vi "Vertical Profile.vi"(5 "Vert.Z-Locations":dbl[](array[numeric])=[12.7, 19.05, 25.4], 6 "Averaging time (min)":dbl, 7 "Lat.Coords":T1={"X"=-3390.0, "Y"=-113.0, "Z"=780.0, "Name"="Anemo1", "Spacing"=enum."Specified", "start"=780.0, "end"=780.0, "NumPts"=780.0, "Specified Locns"=[]}, 9 "Direction":enum16{"Forward", "Reverse"}(ring), 10 "Tunnel Speed":dbl, 11 "Input Task Array":T2[](array[typedef]) {"Carrier_2 Q (l/min)" format="%#.2f"; "Row Duration (mins)" format="%#.1f"; "Row No" min=0; "Trace Gas Concentration (%)" min=0.0 format="%#_4f"; "Carrier_1 Q (l/min)" format="%#.2f"; "Tunnel Speed" format="%#.2f"; "Start X" format="%#.2f"; "Start Y" format="%#.2f"; "Start Z" format="%#.2f"; "End X" format="%#.2f"; "End Y" format="%#.2f"; "End Z" format="%#.2f"; "Averaging time (min)" min=0.0 format="%#.2f"}) -> (3 "Output Task Array":T2[](array[typedef]) {"Carrier_2 Q (l/min)" format="%#.2f"; "Row Duration (mins)" format="%#.1f"; "Row No" min=0; "Trace Gas Concentration (%)" min=0.0 format="%#_4f"; "Carrier_1 Q (l/min)" format="%#.2f"; "Tunnel Speed" format="%#.2f"; "Start X" format="%#.2f"; "Start Y" format="%#.2f"; "Start Z" format="%#.2f"; "End X" format="%#.2f"; "End Y" format="%#.2f"; "End Z" format="%#.2f"; "Averaging time (min)" min=0.0 format="%#.2f"})   [LabVIEW 2015]
uses:
  RowTemplate.ctl
  Anemometry Sub Vis/Gen Trav/Spacing.ctl
  Anemometry Sub Vis/Controls/Multi_run_mode.ctl
  MRCMDFBGlobal.vi
  Set ADAM Ch.vi
panel:
  out "dz":dbl
  # "X           Y            Z"
  # "Start"
  # "End"
  # "X           Y            Z"
  # "Start"
  # "End"
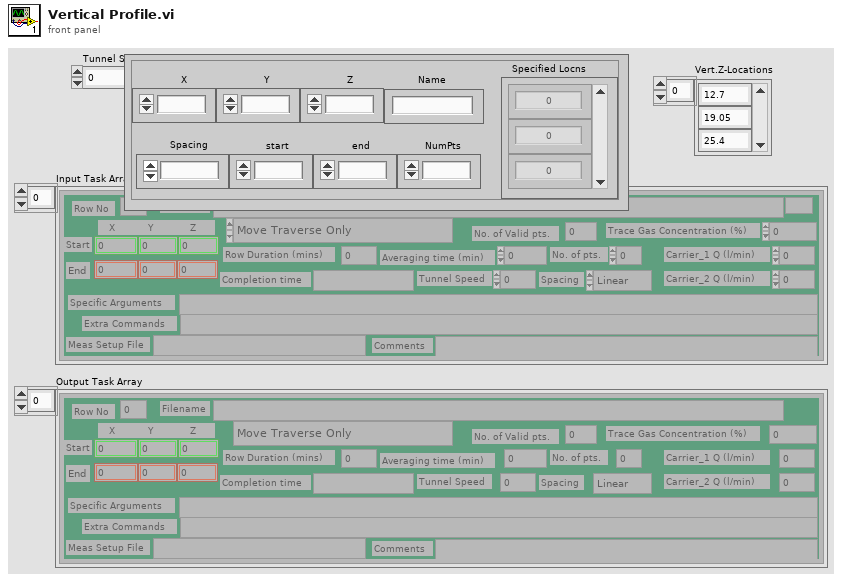
[diagram p1: front panel]
types:
  T1 = cluster{"X":dbl, "Y":dbl, "Z":dbl, "Name":string, "Spacing":enum16{"Linear", "Log", "Gauss", "Specified", "N/A"}, "start":dbl, "end":dbl, "NumPts":dbl, "Specified Locns":dbl[]}
  T2 = typedef "RowTemplate.ctl" = cluster{"Start X":sgl, "Start Y":sgl, "Start Z":sgl, "End X":sgl, "End Y":sgl, "End Z":sgl, "No. of pts.":i32, "Spacing":T3, "Filename":path, "Tunnel Speed":dbl, "Averaging time (min)":dbl, "Extra Commands":string, "Carrier_1 Q (l/min)":dbl, "Carrier_2 Q (l/min)":dbl, "Trace Gas Concentration (%)":dbl, "Specific Arguments":string, "Comments":string, "Row No":i32, "Row Type Selector":T4, "Completion time":string, "Row Duration (mins)":dbl, "No. of Valid pts.":i32, "Meas Setup File":string}
  T3 = typedef "Spacing.ctl" = enum16{"Linear", "Log", "Gauss", "Specified", "N/A"}
  T4 = typedef "Multi_run_mode.ctl" = enum16{"Move Traverse Only", "Set Tunnel Speed Only", "Set Source Only", "Set Measurement Conditions", "Single Measurement", "Vertical Profile", "Lateral Profile", "Longitudinal Profile", "Explore Volume", "Multi-Axis Profile", "Auto Calibrate", "Meas Fast FID Bkgnd", "Check Beam Power", "Scanning Valve Measurement", "Run VI Named:", "Set ADAM Ch", "Wait (minutes)", "Send Message", "Synchronize With:", "Fall Back to this Row", "Turn Off Row Repeating", "Blank Row", "Traverse 3D Volume"}
  T5 = cluster{"Start X":sgl, "Start Y":sgl, "Start Z":sgl, "End X":sgl, "End Y":sgl, "End Z":sgl, "No. of pts.":i32, "Spacing":T3, "Filename":path, "Tunnel Speed":dbl, "Averaging time (min)":dbl, "Extra Commands":string, "Carrier_1 Q (l/min)":dbl, "Carrier_2 Q (l/min)":dbl, "Trace Gas Concentration (%)":dbl, "Specific Arguments":string, "Comments":string, "Row No":i32, "Row Type Selector":T4, "Completion time":string, "Row Duration (mins)":dbl, "No. of Valid pts.":i32, "Meas Setup File":string}[]
  T6 = cluster{"Start X":sgl, "Start Y":sgl, "Start Z":sgl, "End X":sgl, "End Y":sgl, "End Z":sgl, "No. of pts.":i32, "Spacing":T3, "Filename":path, "Tunnel Speed":dbl, "Averaging time (min)":dbl, "Extra Commands":string, "Carrier_1 Q (l/min)":dbl, "Carrier_2 Q (l/min)":dbl, "Trace Gas Concentration (%)":dbl, "Specific Arguments":string, "Comments":string, "Row No":i32, "Row Type Selector":T4, "Completion time":string, "Row Duration (mins)":dbl, "No. of Valid pts.":i32, "Meas Setup File":string}
  T7 = typedef "CorrectionsCluster.ctl" = cluster{"Use Height Corrections":bool, "TT.Azimuths":dbl[], "Z.HeightCorrs":dbl[][], "Corrections from File":bool, "Height Survey Filepaths":path[]}
  T8 = cluster{"Azimuth Array Index":u32, "Vert Prof Array Index":u32, "Lat Prof Array Index":u32, "Long Prof Array Index":u32}
  T9 = enum16{"Linear", "Log", "Gauss", "Specified", "N/A"}
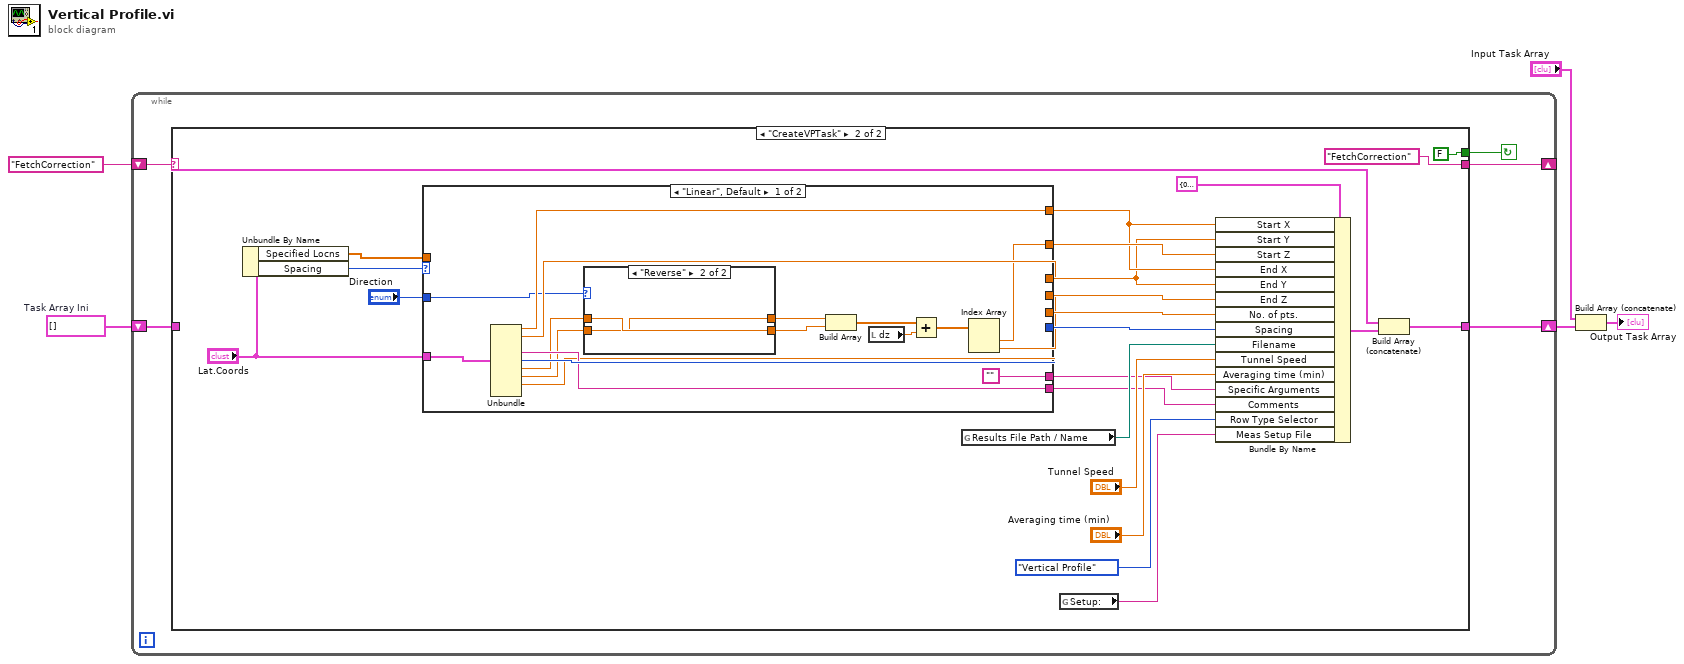
[diagram p0: block diagram]
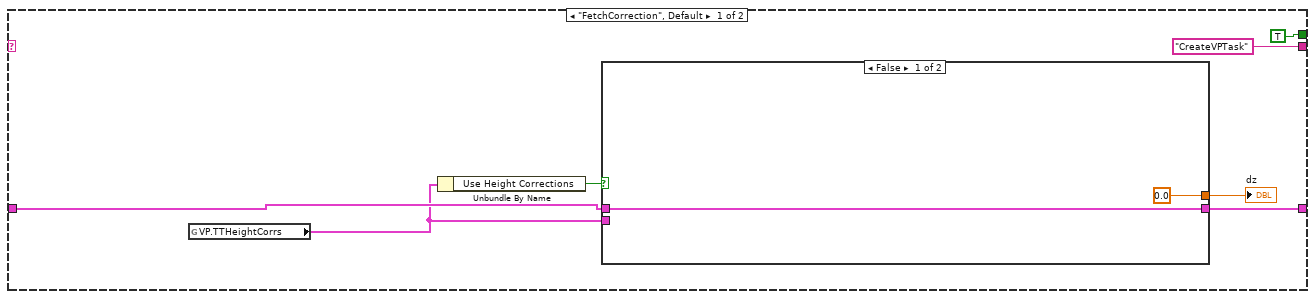
[diagram p2: hidden frame]
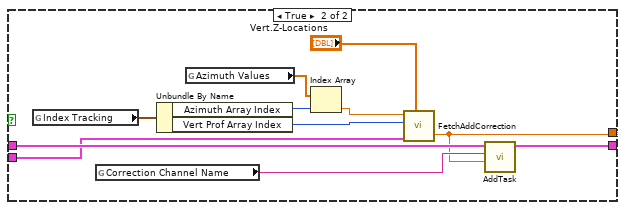
[diagram p3: hidden frame]
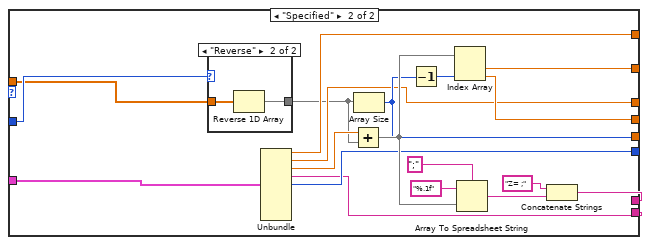
[diagram p5: hidden frame]
diagram:
  w1 = T5 []  # Task Array Ini
  n1 = while {
    shift-right: [w6] -> _
    shift-left: "FetchCorrection" -> [w9]
    shift-right: [w10] -> w3
    shift-left: w1 -> [w8]
    stop <- w7 continue-if-true
    n2 = case shown="\"CreateVPTask\"" w9 {
      tunnel: [w15 w41] -> w10
      tunnel: ["CreateVPTask" "FetchCorrection"] -> w6
      tunnel: w8 -> [w16 w40]
      tunnel: [TRUE FALSE] -> w7
      frame "FetchCorrection", Default {
        n3 = global read "MRCMDFBGlobal.vi" "VP.TTHeightCorrs"() -> (w13:T7)
        n4 = Unbundle By Name(w13) -> ("Use Height Corrections"=w12:bool)
        n5 = case shown="False" w12 {
          tunnel: w16 -> [w19 w27]
          tunnel: [w19 w26] -> w15
          tunnel: w13 -> [_ w21]
          tunnel: [0.0 ("dz") w20] -> w11
          frame False {
          }
          frame True {
            n6 = global read "MRCMDFBGlobal.vi" "Index Tracking"() -> (w30:T8)
            n7 = global read "MRCMDFBGlobal.vi" "Correction Channel Name"() -> (w28:string)
            n8 = Unbundle By Name(w30) -> ("Azimuth Array Index"=w23:u32, "Vert Prof Array Index"=w29:u32)
            n9 = global read "MRCMDFBGlobal.vi" "Azimuth Values"() -> (w24:dbl[])
            n10 = Index Array(array=w24, index=w23) -> (element=w22:dbl)
            n11 = call "FetchAddCorrection.vi"("Azimuth Value"=w22, "Vert Prof Array Index"=w29, "VP.TTHeightCorrs"=w21, "Vert.Z-Locations"="Vert.Z-Locations") -> ("dz"=w20:dbl)  [unwired: 1 in, 1 out]
            n12 = call-poly "AddTask.vi"("Value"=w20, "ADAM:Channel:Name"=w28, "Input Task Array"=w27) -> ("Output Task Array"=w26:T2[])  [unwired: 8 in]
          }
        }
        "dz" <- w11
      }
      frame "CreateVPTask" {
        n13 = Unbundle By Name("Lat.Coords") -> ("Specified Locns"=w31:dbl[], "Spacing"=w38:T9)
        n14 = case shown="\"Linear\", Default" w38 {
          tunnel: ["" w87] -> w47
          tunnel: [w65 w86] -> w46
          tunnel: [w60 w85] -> w45
          tunnel: [w59 w84] -> w44
          tunnel: "Lat.Coords" -> [w70 w83]
          tunnel: [w69 w79] -> w37
          tunnel: [w68 w78] -> w36
          tunnel: [w67 w82] -> w35
          tunnel: [w66 w81] -> w34
          tunnel: "Direction" -> [w58 w77]
          tunnel: w31 -> [_ w75]
          frame "Linear", Default {
            n15 = Unbundle(w70) -> ("X"=w67:dbl, "Y"=w66:dbl, "Name"=w68:string, "Spacing"=w69:T9, "start"=w57:dbl, "end"=w55:dbl, "NumPts"=w65:dbl)  [unwired: 2 out]
            n16 = case shown="\"Reverse\"" w58 {
              tunnel: w57 -> [w72 w74]
              tunnel: [w72 w73] -> w56
              tunnel: w55 -> [w71 w73]
              tunnel: [w71 w74] -> w54
              frame "Forward", Default {
              }
              frame "Reverse" {
              }
            }
            n17 = Build Array(w56, w54) -> (w62:dbl[])
            n18 = local read "dz"() -> (w63:dbl)
            n19 = Add(x=w62, y=w63) -> (x+y=w61:dbl[])
            n20 = Index Array(array=w61) -> (element #1=w60:dbl, element #2=w59:dbl)  [unwired: 2 in]
          }
          frame "Specified" {
            n21 = case shown="\"Reverse\"" w77 {
              tunnel: [w94 w95] -> w76
              tunnel: w75 -> [w94 w96]
              frame "Forward", Default {
              }
              frame "Reverse" {
                n22 = Reverse 1D Array(array=w96) -> (reversed array=w95:dbl[])
              }
            }
            n23 = Unbundle(w83) -> ("X"=w82:dbl, "Y"=w81:dbl, "Z"=w80:dbl, "Name"=w78:string, "Spacing"=w79:T9)  [unwired: 4 out]
            n24 = Add(x=w80, y=w76) -> (x+y=w93:dbl[])
            n25 = Array Size(array=w76) -> (size(s)=w86:i32)
            n26 = Decrement(x=w86) -> (x-1=w90:i32)
            n27 = Index Array(array=w93, index #2=w90) -> (element #1=w85:dbl, element #2=w84:dbl)  [unwired: 1 in]
            n28 = Array To Spreadsheet String(delimiter (Tab)=";", array=w93, 3:"%.1f" ("format string")) -> (spreadsheet string=w91:string)
            n29 = Concatenate Strings("Z= ;", w91) -> (w87:string)
          }
        }
        n30 = global read "MRCMDFBGlobal.vi" "Results File Path / Name"() -> (w48:path)
        n31 = global read "MRCMDFBGlobal.vi" "Setup:"() -> (w49:string)
        n32 = Bundle By Name(cluster=T6 {"Start X"=0.0, "Start Y"=0.0, "Start Z"=0.0, "End X"=0.0, "End Y"=0.0, "End Z"=0.0, "No. of pts."=0, "Spacing"=enum."Linear", "Filename"=path "", "Tunnel Speed"=0.0, "Averaging time (min)"=0.0, "Extra Commands"="", "Carrier_1 Q (l/min)"=0.0, "Carrier_2 Q (l/min)"=0.0, "Trace Gas Concentration (%)"=0.0, "Specific Arguments"="", "Comments"="", "Row No"=0, "Row Type Selector"=enum."Move Traverse Only", "Completion time"="", "Row Duration (mins)"=0.0, "No. of Valid pts."=0, "Meas Setup File"=""} ("RowTemplateConst"), "Start X"=w35, "Start Y"=w34, "Start Z"=w45, "End X"=w35, "End Y"=w34, "End Z"=w44, "No. of pts."=w46, "Spacing"=w37, "Filename"=w48, "Tunnel Speed"="Tunnel Speed", "Averaging time (min)"="Averaging time (min)", "Specific Arguments"=w47, "Comments"=w36, "Row Type Selector"=Multi_run_mode."Vertical Profile", "Meas Setup File"=w49) -> (w42:T6)
        n33 = Build Array (concatenate)(w40, w42) -> (w41:T2[])
      }
    }
  }
  n34 = Build Array (concatenate)("Input Task Array", w3) -> (→"Output Task Array":T2[])
